vi "TEMP_SCAN.vi"(8 "error in (no error)":errorcluster, 9 "Boolean":bool, 10 "ScanQ in":refnum<queue>, 11 "SweepQ in":refnum<queue>) -> (0 "error out":errorcluster, 2 "ScanQ out":refnum<queue>, 3 "SweepQ out":refnum<queue>)   [LabVIEW 2025]
uses:
  Desktop/STM-Auto-Project/QMH CTLS/Scan_Params (QMH).ctl
  TEMP_SWEEPER.ctl
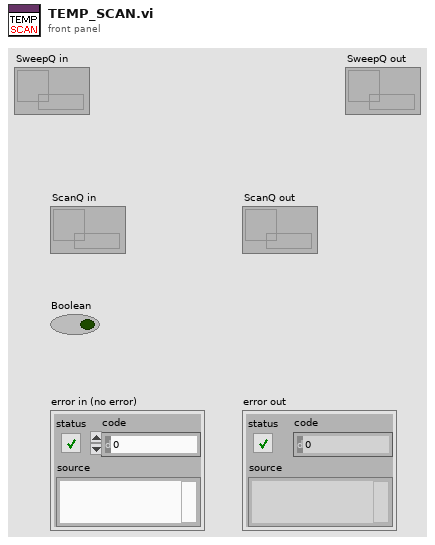
[diagram p1: front panel]
types:
  T1 = enum16{"1. BIAS", "2. INIT_SCAN", "3. SCAN_IDLE", "4. INTER_SCAN", "5. NEW_COORDS_&_FRAME", "6. FINAL_SCAN", "7. POLL BIAS ", "8. Z-CONT.", "9. STOP"}
  T2 = enum16{"SET TEMP", "SWEEP IDLE", "NEXT TEMP", "SWEEP DONE"}
  T3 = typedef "TEMP_SWEEPER.ctl" = cluster{"Temps(K)":dbl[], "Sweep States":enum16{"SET TEMP", "SWEEP IDLE", "NEXT TEMP", "SWEEP DONE"}}
  T4 = typedef "Scan_Params (QMH).ctl" = cluster{"Setpoint (I)":dbl[], "Bias (V)":dbl[], "Number of scans":u8, "Port number (3364)":u32, "Avoid zero threshold (V)":dbl, "Current State":enum16{"1. BIAS", "2. INIT_SCAN", "3. SCAN_IDLE", "4. INTER_SCAN", "5. NEW_COORDS_&_FRAME", "6. FINAL_SCAN", "7. POLL BIAS ", "8. Z-CONT.", "9. STOP"}}
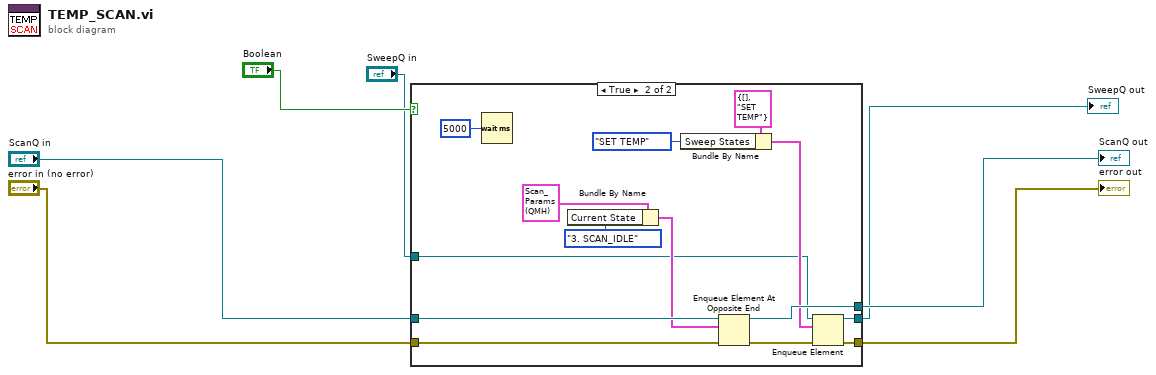
[diagram p0: block diagram]
diagram:
  n1 = case shown="True" "Boolean" {
    tunnel: [w10 w20] -> w6
    tunnel: "error in (no error)" -> [w9 w19]
    tunnel: "ScanQ in" -> [w10 w22]
    tunnel: [w9 w23] -> w7
    tunnel: "SweepQ in" -> [w8 w14]
    tunnel: [w8 w13] -> w1
    frame False {
    }
    frame True {
      n2 = Wait (ms)(milliseconds to wait=u32 5000) -> ()  [unwired: 1 out]
      n3 = Bundle By Name(cluster=T4 {"Setpoint (I)"=[], "Bias (V)"=[], "Number of scans"=1, "Port number (3364)"=3364, "Avoid zero threshold (V)"=0.004999999888241291, "Current State"=enum."1. BIAS"} ("element"), "Current State"=T1."3. SCAN_IDLE") -> (w17:T4)
      n4 = Bundle By Name(cluster=T3 {"Temps(K)"=[], "Sweep States"=enum."SET TEMP"} ("Temp and Field Range"), "Sweep States"=T2."SET TEMP") -> (w15:T3)
      n5 = Enqueue Element At Opposite End(queue=w22, element=w17, error in (no error)=w19) -> (queue out=w20:refnum<queue>, error out=w18:errorcluster)  [unwired: 1 in, 1 out]
      n6 = Enqueue Element(queue=w14, element=w15, error in (no error)=w18) -> (queue out=w13:refnum<queue>, error out=w23:errorcluster)  [unwired: 1 in, 1 out]
    }
  }
  "error out" <- w7
  "ScanQ out" <- w6
  "SweepQ out" <- w1
